vi "Do.vi"(8 "error in (no error)":errorcluster, 10 "Actor in":refnum<class "Actor.lvclass">, 11 "Set Calculation State Msg":refnum<class "Set Calculation State Msg.lvclass">) -> (0 "error out":errorcluster, 2 "Actor out":refnum<class "Actor.lvclass">)   [LabVIEW 2020, in "CPU FFT Calculator.lvlib" / "Set Calculation State Msg.lvclass"]
doc: "This VI delivers the message to the actor by calling the appropriate method(s) on the actor."
uses:
  Set Calculation State Msg.lvclass
  <vilib>/ActorFramework/Actor/Actor.lvclass
  CPU FFT Calculator/CPU FFT Calculator.lvclass
  C:/Program Files/National Instruments/LabVIEW 2026/vi.lib/ActorFramework/Actor/Actor.lvclass
  34700b1e-4b1b-4205-ab4b-28631ba2a4c6.vi
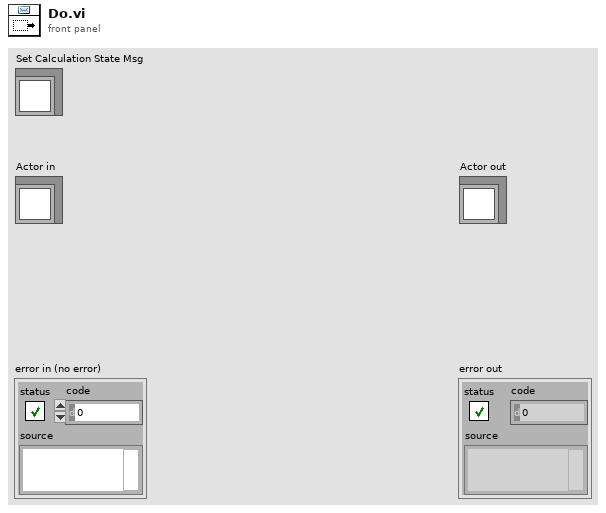
[diagram p1: front panel]
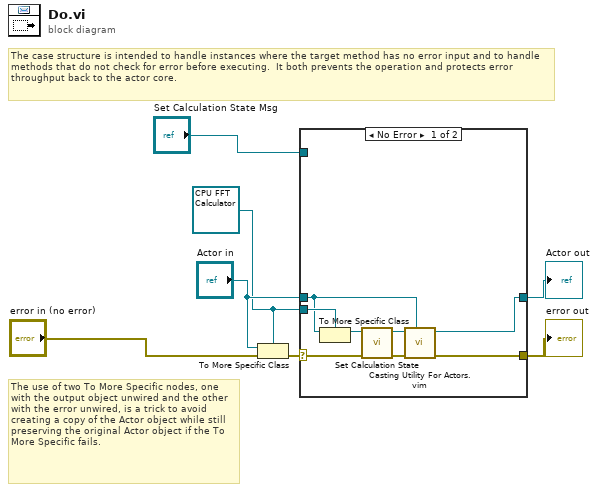
[diagram p0: block diagram]
diagram:
  w2 = refnum<class "CPU FFT Calculator.lvclass"> refnum ("Actor in")
  # "The use of two To More Specific nodes, one with the output object unwired and the other with the error unwired, is a trick to avoid creating a copy of the Actor object while still preserving the original Actor object if the To More Specific fails."
  # "The case structure is intended to handle instances where the target method has no error input and to handle methods that do not check for error before executing.  It both prevents the operation and protects error throughput back to the actor core."
  n1 = To More Specific Class(target class=w2, reference="Actor in", error in="error in (no error)") -> (error out=w6:errorcluster)  [unwired: 1 out]
  n2 = case shown="No Error" w6 {
    selector: w6 -> [w15 w17]
    tunnel: [w9 w17] -> w5
    tunnel: [w8 w16] -> w4
    tunnel: "Actor in" -> [w12 w16]
    tunnel: w2 -> [w13 _]
    tunnel: "Set Calculation State Msg" -> [_ _]
    frame No Error {
      n3 = To More Specific Class(target class=w13, reference=w12) -> (specific class reference=w14:refnum<class "CPU FFT Calculator.lvclass">)  [unwired: 1 in, 1 out]
      n4 = call-dynamic "Set Calculation State.vi"("error in (no error)"=w15, "CPU FFT Calculator in"=w14) -> ("error out"=w10:errorcluster, "CPU FFT Calculator out"=w11:refnum<class "CPU FFT Calculator.lvclass">)  [unwired: 8 in]
      n5 = call "Casting Utility For Actors.vim"("type"=w12, "error in (no error)"=w10, "Actor in"=w11) -> ("error out"=w9:errorcluster, "Actor out"=w8:refnum<class "Actor.lvclass">)  [unwired: 7 in]
    }
    frame Error {
      # "If type check fails, pass the original object out again."
    }
  }
  "error out" <- w5
  "Actor out" <- w4
